vi "Visa_dso.vi"() -> ()   [LabVIEW 2018]
panel:
  in  "Tab Control":enum32{"Page 1", "Page 2"}(tab)
  out "error out":errorcluster
  out "read buffer":string
  in  "VISA resource name":refnum<visa-resource-name>
  in  "write buffer":string
  in  "File Directory":path=path "E:/Ankur/Labview/Automation/Data/Exp1"
  out "Output Filename":path
  out "Output Directory":path
  in  "Filename":string
  in  "byte count":u32
  out "return count":u32
  out "error out 2":errorcluster
  out "event":refnum<visa-resource-name>
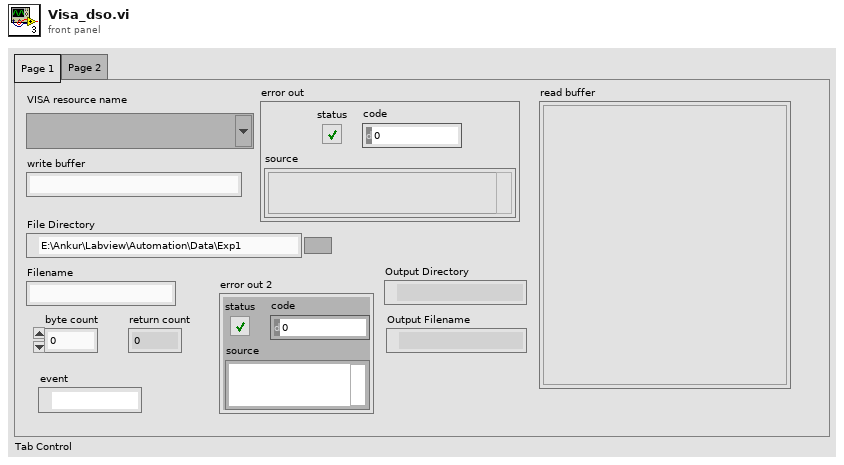
[diagram p1: front panel]
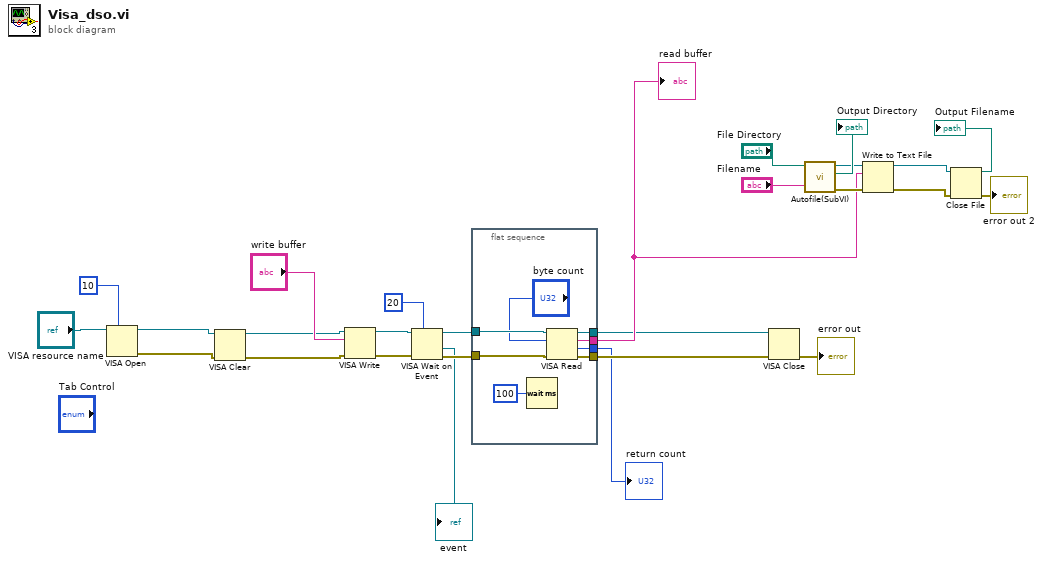
[diagram p0: block diagram]
diagram:
  n1 = VISA Open(timeout (0)=u32 10 ("VISA Open timeout (0)"), VISA resource name="VISA resource name") -> (VISA resource name=w14:refnum<visa-resource-name>, error out=w13:errorcluster)  [unwired: 3 in]
  n2 = VISA Clear(VISA resource name=w14, error in (no error)=w13) -> (VISA resource name out=w12:refnum<visa-resource-name>, error out=w11:errorcluster)
  n3 = VISA Write(VISA resource name=w12, write buffer="write buffer", error in (no error)=w11) -> (VISA resource name out=w6:refnum<visa-resource-name>, error out=w5:errorcluster)  [unwired: 1 out]
  n4 = VISA Wait on Event(7:u32 20 ("timeout (0)"), 8:w5, 11:w6) -> (0:w3:errorcluster, 1:→"event":refnum<visa-resource-name>, 3:w4:refnum<visa-resource-name>)  [unwired: 2 in, 1 out]
  n5 = flat-sequence {
    tunnel: w4 -> [w35]
    tunnel: w3 -> [w34]
    tunnel: [w32] -> w17
    tunnel: [w31] -> w9
    tunnel: [w30] -> w8
    tunnel: [w29] -> w7
    frame #0 {
      n6 = Wait (ms)(milliseconds to wait=u32 100) -> ()  [unwired: 1 out]
      n7 = VISA Read(VISA resource name=w35, byte count="byte count", error in (no error)=w34) -> (VISA resource name out=w31:refnum<visa-resource-name>, read buffer=w32:string, return count=w29:u32, error out=w30:errorcluster)
    }
  }
  n8 = VISA Close(VISA resource name=w9, error in (no error)=w8) -> (error out=→"error out":errorcluster)
  n9 = call "Autofile(SubVI).vi"("Filename"="Filename", "File Directory"="File Directory") -> ("error out"=w20:errorcluster, "Output Directory"=→"Output Directory":path, "Byte Stream File out"=w21:refnum<file>)  [unwired: 7 in]
  n10 = Write to Text File(file (use dialog)=w21, text=w17, error in=w20) -> (refnum out=w18:refnum<file>, error out=w19:errorcluster)  [unwired: 1 in, 1 out]
  n11 = Close File(refnum=w18, error in=w19) -> (path=→"Output Filename":path, error out=→"error out 2":errorcluster)
  "read buffer" <- w17
  "return count" <- w7
